vi "AOC_FloodSearch.vi"(6 "4 (T) or 8 (F)":bool, 7 "AllowPixelsOnBorder(True)":bool=TRUE, 8 "error in (no error)":errorcluster, 9 "StopWhenLength>":i32, 10 "Start Position":cluster{"x":i32, "y":i32}={"x"=5, "y"=5}, 11 "DataIn":bool[][](array[boolean])=[[FALSE, FALSE, FALSE, FALSE, FALSE, FALSE, FALSE, FALSE, FALSE, FALSE, FALSE], [FALSE, FALSE, FALSE, FALSE, FALSE, FALSE, FALSE, FALSE, FALSE, FALSE, FALSE], [FALSE, FALSE, FALSE, FALSE, FALSE, FALSE, FALSE, FALSE, FALSE, FALSE, FALSE], [FALSE, FALSE, FALSE, FALSE, FALSE, FALSE, FALSE, FALSE, FALSE, FALSE, FALSE], [FALSE, FALSE, FALSE, FALSE, FALSE, FALSE, FALSE, FALSE, FALSE, FALSE, FALSE], [FALSE, FALSE, FALSE, FALSE, FALSE, FALSE, FALSE, FALSE, FALSE, FALSE, FALSE], [FALSE, FALSE, FALSE, FALSE, FALSE, FALSE, FALSE, FALSE, FALSE, FALSE, FALSE], [FALSE, FALSE, FALSE, FALSE, FALSE, FALSE, FALSE, FALSE, FALSE, FALSE, FALSE], [FALSE, FALSE, FALSE, FALSE, FALSE, FALSE, FALSE, FALSE, FALSE, FALSE, FALSE]]) -> (0 "error out":errorcluster, 1 "Length":dbl, 2 "LengthFound":bool, 3 "PixelsFound":cluster{"x":i32, "y":i32}[](array[cluster]))   [LabVIEW 2023]
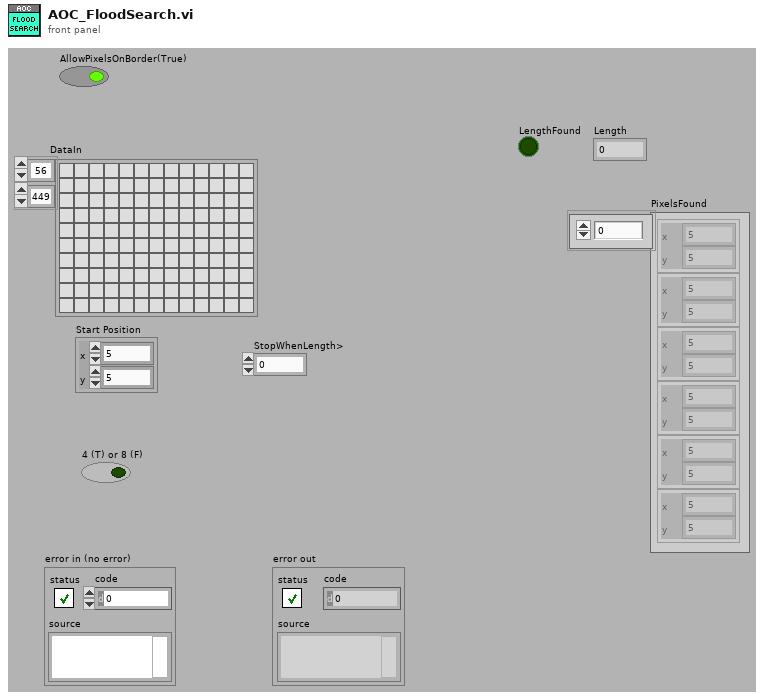
[diagram p1: front panel]
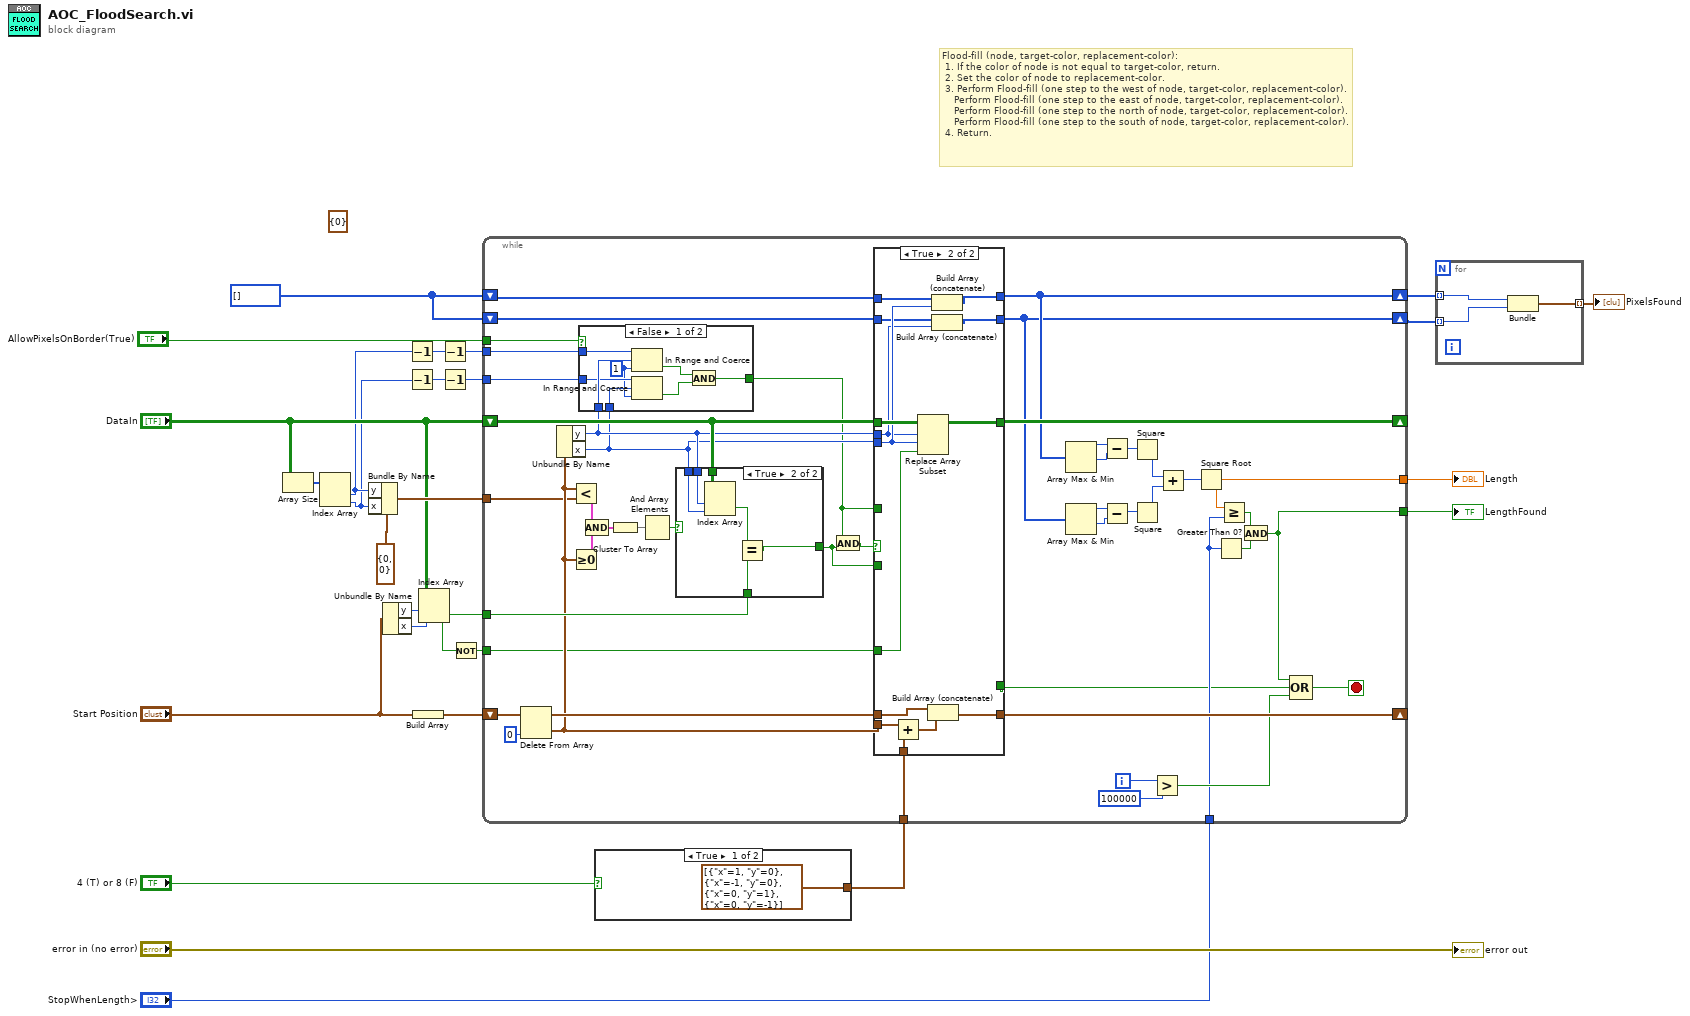
[diagram p0: block diagram]
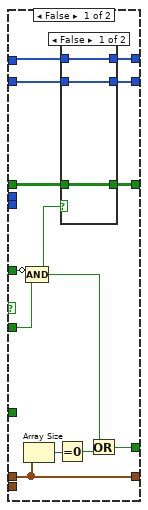
[diagram p2: hidden frame]
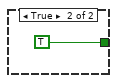
[diagram p4: hidden frame]
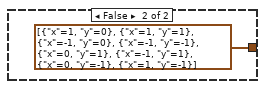
[diagram p6: hidden frame]
diagram:
  (unwired) cluster{"x":i32} {"x"=0}
  w17 = i32[] []
  # "Flood-fill (node, target-color, replacement-color):\n 1. If the color of node is not equal to target-color, return.\n 2. Set the color of node to replacement-color.\n 3. Perform Flood-fill (one step to the west of node, target-color, replacement-color).\n    Perform Flood-fill (one step to the east of node, target-color, replacement-color).\n    Perform Flood-fill (one step to the north of node, target-color, replacement-color).\n    Perform Flood-fill (one step to the south of node, target-color, replacement-color).\n 4. Return."
  n1 = Array Size(array="DataIn") -> (size(s)=w24:i32[])
  n2 = Index Array(array=w24) -> (element #1=w6:i32, element #2=w3:i32)  [unwired: 2 in]
  n3 = Bundle By Name(cluster=cluster{"x":i32, "y":i32} {"x"=0, "y"=0} ("input cluster"), "y"=w6, "x"=w3) -> (w23:cluster{"x":i32, "y":i32})
  n4 = Unbundle By Name("Start Position") -> ("y"=w19:i32, "x"=w18:i32)
  n5 = Decrement(x=w6) -> (x-1=w5:i32)
  n6 = Decrement(x=w3) -> (x-1=w2:i32)
  n7 = Build Array("Start Position") -> (w20:cluster{"x":i32, "y":i32}[])
  n8 = Index Array(array="DataIn", index (row)=w19, index (col)=w18) -> (element=w10:bool)
  n9 = Decrement(x=w5) -> (x-1=w4:i32)
  n10 = Decrement(x=w2) -> (x-1=w1:i32)
  n11 = Not(x=w10) -> (.not. x?=w9:bool)
  n12 = case shown="True" "4 (T) or 8 (F)" {
    tunnel: [cluster{"x":i32, "y":i32}[] [{"x"=1, "y"=0}, {"x"=-1, "y"=0}, {"x"=0, "y"=1}, {"x"=0, "y"=-1}] cluster{"x":i32, "y":i32}[] [{"x"=1, "y"=0}, {"x"=1, "y"=1}, {"x"=-1, "y"=0}, {"x"=-1, "y"=-1}, {"x"=0, "y"=1}, {"x"=-1, "y"=1}, {"x"=0, "y"=-1}, {"x"=1, "y"=-1}]] -> w22
    frame True {
    }
    frame False {
    }
  }
  n13 = while {
    shift-right: [w76] -> _
    shift-left: "DataIn" -> [w75]
    shift-right: [w74] -> _
    shift-left: w20 -> [w73]
    tunnel: w10 -> [w70]
    tunnel: w23 -> [w66]
    tunnel: w22 -> [w62]
    shift-right: [w55] -> w14
    shift-left: w17 -> [w61]
    shift-right: [w54] -> w13
    shift-left: w17 -> [w56]
    tunnel: "StopWhenLength>" -> [w52]
    tunnel: [w51] -> w15
    tunnel: [w53] -> w12
    tunnel: w9 -> [w50]
    tunnel: "AllowPixelsOnBorder(True)" -> [w49]
    tunnel: w4 -> [w47]
    tunnel: w1 -> [w46]
    i -> [w60]
    stop <- w57 stop-if-true
    n14 = Delete From Array(array=w73, index=0) -> (deleted portion=w67:cluster{"x":i32, "y":i32}, array with subset deleted=w72:cluster{"x":i32, "y":i32}[])  [unwired: 1 in]
    n15 = Unbundle By Name(w67) -> ("y"=w48:i32, "x"=w45:i32)
    n16 = Less?(x=w67, y=w66) -> (x < y?=w69:cluster{"x":bool, "y":bool})
    n17 = Greater Or Equal To 0?(x=w67) -> (x >= 0?=w68:cluster{"x":bool, "y":bool})
    n18 = case shown="False" w49 {
      tunnel: [w108 TRUE] -> w31
      tunnel: w48 -> [w114 _]
      tunnel: w47 -> [w113 _]
      tunnel: w46 -> [w112 _]
      tunnel: w45 -> [w111 _]
      frame False {
        w110 = 1 ("lower limit")
        n19 = In Range and Coerce(upper limit=w113, x=w114, lower limit=w110) -> (In Range?=w107:bool)  [unwired: 1 out]
        n20 = In Range and Coerce(upper limit=w112, x=w111, lower limit=w110) -> (In Range?=w109:bool)  [unwired: 1 out]
        n21 = And(x=w107, y=w109) -> (x .and. y?=w108:bool)
      }
      frame True {
      }
    }
    n22 = Compound Arithmetic op=AND(w69, w68) -> (w65:cluster{"x":bool, "y":bool})
    n23 = Cluster To Array(cluster=w65) -> (array=w64:bool[])
    n24 = And Array Elements(Boolean array=w64) -> (logical AND=w63:bool)
    n25 = case shown="True" w63 {
      selector: w63 -> [w116 _]
      tunnel: w75 -> [_ w122]
      tunnel: [w116 w117] -> w30
      tunnel: w70 -> [_ w121]
      tunnel: w48 -> [_ w120]
      tunnel: w45 -> [_ w119]
      frame False {
      }
      frame True {
        n26 = Index Array(array=w122, index (row)=w120, index (col)=w119) -> (element=w118:bool)
        n27 = Equal?(x=w118, y=w121) -> (x = y?=w117:bool)
      }
    }
    n28 = And(x=w31, y=w30) -> (x .and. y?=w32:bool)
    n29 = case shown="True" w32 {
      tunnel: w75 -> [w82 w106]
      tunnel: [w79 w105] -> w76
      tunnel: w45 -> [_ w97]
      tunnel: w48 -> [_ w95]
      tunnel: w67 -> [_ w102]
      tunnel: w72 -> [w88 w104]
      tunnel: [w88 w103] -> w74
      tunnel: w62 -> [_ w101]
      tunnel: [w85 _] -> w44
      tunnel: w61 -> [w80 w99]
      tunnel: [w77 w98] -> w55
      tunnel: w56 -> [w81 w96]
      tunnel: [w78 w94] -> w54
      tunnel: w50 -> [_ w93]
      tunnel: w31 -> [w86 _]
      tunnel: w30 -> [w84 _]
      frame False {
        n30 = Array Size(array=w88) -> (size(s)=w89:i32)
        n31 = Compound Arithmetic op=AND(invert w86, w84) -> (w83:bool)
        n32 = Equal To 0?(x=w89) -> (x = 0?=w87:bool)
        n33 = case shown="False" w83 {
          tunnel: w82 -> [w92 _]
          tunnel: w81 -> [w91 _]
          tunnel: w80 -> [w90 _]
          tunnel: [w92 _] -> w79
          tunnel: [w91 _] -> w78
          tunnel: [w90 _] -> w77
          frame False {
          }
          frame True {
          }
        }
        n34 = Or(x=w83, y=w87) -> (x .or. y?=w85:bool)
      }
      frame True {
        n35 = Add(x=w102, y=w101) -> (x+y=w100:cluster{"x":i32, "y":i32}[])
        n36 = Replace Array Subset(array=w106, new element=w93, index (row)=w95, index (col)=w97) -> (w105:bool[][])
        n37 = Build Array (concatenate)(w104, w100) -> (w103:cluster{"x":i32, "y":i32}[])
        n38 = Build Array (concatenate)(w99, w97) -> (w98:i32[])
        n39 = Build Array (concatenate)(w96, w95) -> (w94:i32[])
      }
    }
    n40 = Array Max & Min(array=w55) -> (max value=w43:i32, min value=w42:i32)  [unwired: 2 out]
    n41 = Array Max & Min(array=w54) -> (max value=w41:i32, min value=w40:i32)  [unwired: 2 out]
    n42 = Subtract(x=w43, y=w42) -> (x-y=w39:i32)
    n43 = Subtract(x=w41, y=w40) -> (x-y=w38:i32)
    n44 = Square(x=w39) -> (x^2=w37:i32)
    n45 = Square(x=w38) -> (x^2=w36:i32)
    n46 = Greater?(x=w60, y=100000) -> (0:w58:bool)
    n47 = Add(x=w37, y=w36) -> (x+y=w35:i32)
    n48 = Square Root(x=w35) -> (sqrt(x)=w53:dbl)
    n49 = Greater Than 0?(x=w52) -> (x > 0?=w33:bool)
    n50 = Greater Or Equal?(x=w53, y=w52) -> (x >= y?=w34:bool)
    n51 = And(x=w34, y=w33) -> (x .and. y?=w51:bool)
    n52 = Compound Arithmetic op=OR(w51, w44, w58) -> (w57:bool)
  }
  "LengthFound" <- w15
  "Length" <- w12
  n53 = for {
    tunnel: w14 -> [w125] mode=indexing
    tunnel: w13 -> [w124] mode=indexing
    tunnel: [w123] -> w11 mode=indexing
    n54 = Bundle("y"=w125, "y"=w124) -> (w123:cluster{"y":i32, "y":i32})  [unwired: 1 in]
  }
  "PixelsFound" <- w11
  "error out" <- "error in (no error)"
